vi "Shared_Variable_test_1.vi"() -> ()   [LabVIEW 2016]
panel:
  out "Writing current time":timestamp
  in  "Stop Button":bool
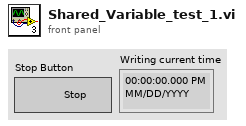
[diagram p1: front panel]
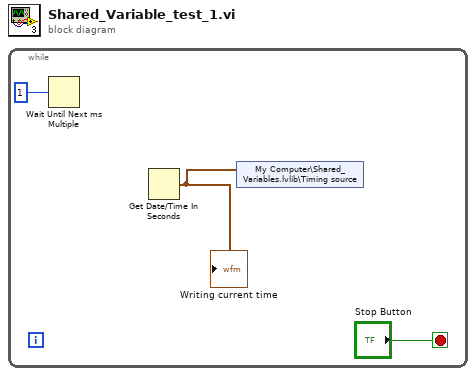
[diagram p0: block diagram]
diagram:
  n1 = while {
    stop <- "Stop Button" stop-if-true
    n2 = Wait Until Next ms Multiple(millisecond multiple=u32 1) -> ()  [unwired: 1 out]
    n3 = Get Date/Time In Seconds() -> (seconds since 1Jan1904=w3:timestamp)
    "Writing current time" <- w3
    n4 = shared-variable "My Computer\\Shared_Variables.lvlib\\Timing source"(w3) -> ()  [unwired: 1 in, 1 out]
  }
